vi "CalcDirection.vi"(8 "error in (no error)":errorcluster, 9 "DirectionY":i8, 10 "DirectionX":i8, 11 "Snake in":refnum<class "Snake.lvclass">) -> (0 "error out":errorcluster, 3 "Snake out":refnum<class "Snake.lvclass">)   [LabVIEW 2019, in "RT_Game.lvlib" / "Snake.lvclass"]
uses:
  Snake.lvclass
  Snake.lvclass/Snake.ctl
  Direction.ctl
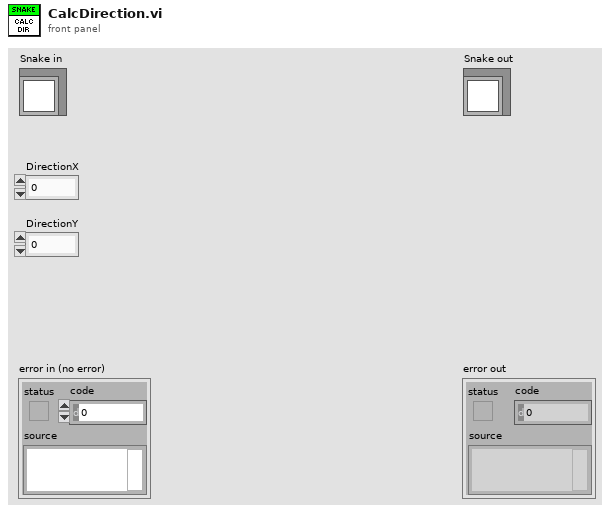
[diagram p1: front panel]
types:
  T1 = typedef "RT_Game.lvlib/Snake.lvclass/Direction.ctl" = enum16{"Up", "Left", "Down", "Right"}
  T2 = typedef "RT_Game.lvlib/Game.lvclass/Coordinate.ctl" = cluster{"x":dbl, "y":dbl}
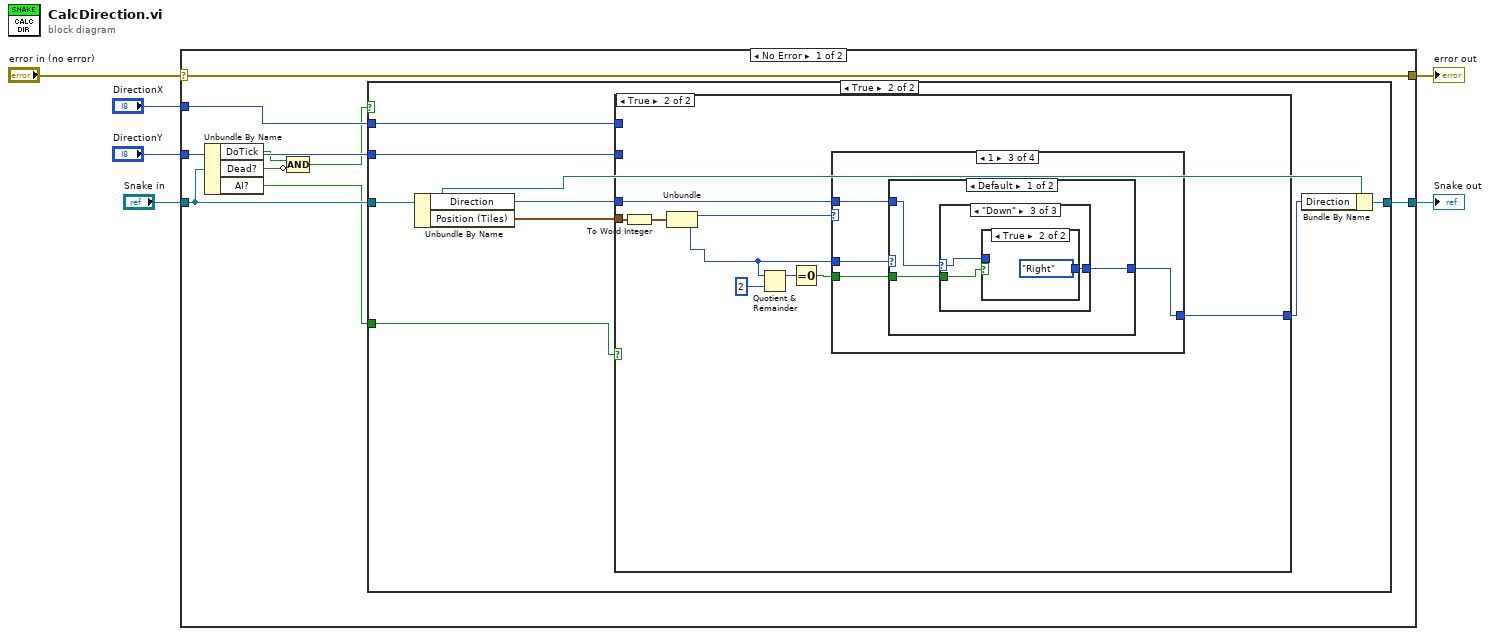
[diagram p0: block diagram]
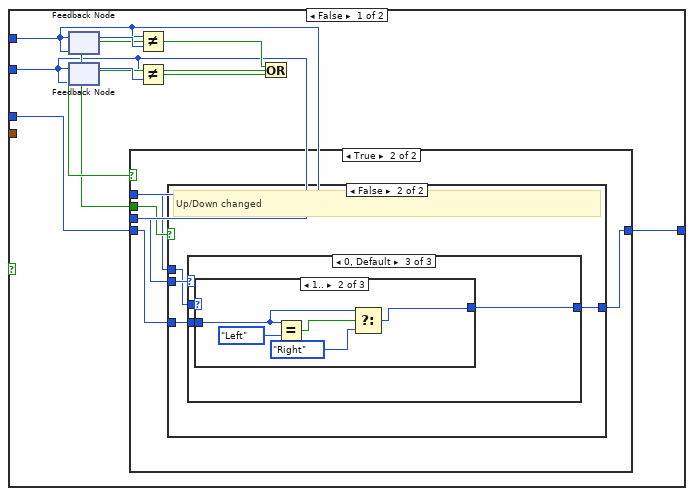
[diagram p3: hidden frame]
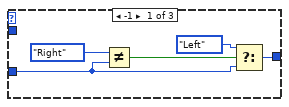
[diagram p6: hidden frame]
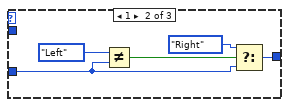
[diagram p7: hidden frame]
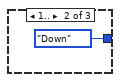
[diagram p8: hidden frame]
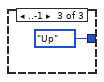
[diagram p9: hidden frame]
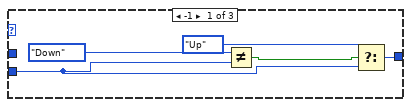
[diagram p10: hidden frame]
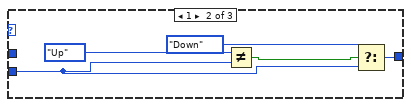
[diagram p11: hidden frame]
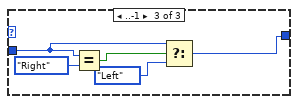
[diagram p13: hidden frame]
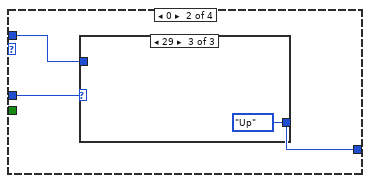
[diagram p15: hidden frame]
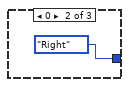
[diagram p17: hidden frame]
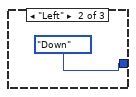
[diagram p19: hidden frame]
diagram:
  n1 = case shown="No Error" "error in (no error)" {
    selector: "error in (no error)" -> [w15 w125]
    tunnel: [w15 w125] -> w5
    tunnel: [w14 w124] -> w3
    tunnel: "Snake in" -> [w11 w124]
    tunnel: "DirectionX" -> [w13 _]
    tunnel: "DirectionY" -> [w12 _]
    frame No Error {
      n2 = Unbundle By Name(w11) -> ("DoTick"=w8:bool, "Dead?"=w10:bool, "AI?"=w7:bool)
      n3 = Compound Arithmetic op=AND(w8, invert w10) -> (w9:bool)
      n4 = case shown="True" w9 {
        tunnel: [w16 w23] -> w14
        tunnel: w13 -> [_ w21]
        tunnel: w12 -> [_ w20]
        tunnel: w11 -> [w16 w19]
        tunnel: w7 -> [_ w18]
        frame False {
        }
        frame True {
          n5 = Unbundle By Name(w19) -> ("Direction"=w24:T1, "Position (Tiles)"=w17:T2)
          n6 = case shown="True" w18 {
            tunnel: w24 -> [w28 w94]
            tunnel: [w27 w93] -> w22
            tunnel: w21 -> [w26 _]
            tunnel: w20 -> [w25 _]
            tunnel: w17 -> [_ w96]
            frame False {
              n7 = feedback #1(w26) -> (w33:i8)
              n8 = feedback-in #1(w26) -> ()
              n9 = feedback #2(w25) -> (w32:i8)
              n10 = feedback-in #2(w25) -> ()
              n11 = Not Equal?(x=w26, y=w33) -> (x != y?=w29:bool)
              n12 = Not Equal?(x=w25, y=w32) -> (x != y?=w31:bool)
              n13 = Or(x=w29, y=w31) -> (x .or. y?=w30:bool)
              n14 = case shown="True" w30 {
                tunnel: w26 -> [_ w38]
                tunnel: w25 -> [_ w35]
                tunnel: w29 -> [_ w39]
                tunnel: w28 -> [w34 w37]
                tunnel: [w34 w36] -> w27
                frame False {
                }
                frame True {
                  n15 = case shown="False" w39 {
                    tunnel: w38 -> [w43 w60]
                    tunnel: w37 -> [w42 w63]
                    tunnel: [w41 w62] -> w36
                    tunnel: w35 -> [w40 w61]
                    frame True {
                      # "Left/Right changed"
                      n16 = case shown="0, Default" w43 {
                        tunnel: [w46 w49 w55] -> w41
                        tunnel: w42 -> [w47 w50 w54]
                        tunnel: w40 -> [_ _ w56]
                        frame -1 {
                          n17 = Not Equal?(x=Direction."Right", y=w47) -> (x != y?=w45:bool)
                          n18 = Select(t=Direction."Left", s=w45, f=w47) -> (s? t:f=w46:T1)
                        }
                        frame 1 {
                          n19 = Not Equal?(x=Direction."Left", y=w50) -> (x != y?=w53:bool)
                          n20 = Select(t=Direction."Right", s=w53, f=w50) -> (s? t:f=w49:T1)
                        }
                        frame 0, Default {
                          n21 = case shown="0, Default" w56 {
                            tunnel: [w57 Direction."Down" ("Direction") Direction."Up" ("Direction")] -> w55
                            tunnel: w54 -> [w57 _ _]
                            frame 0, Default {
                            }
                            frame 1.. {
                            }
                            frame ..-1 {
                            }
                          }
                        }
                      }
                    }
                    frame False {
                      # "Up/Down changed"
                      n22 = case shown="0, Default" w61 {
                        tunnel: [w66 w69 w75] -> w62
                        tunnel: w63 -> [w67 w70 w74]
                        tunnel: w60 -> [_ _ w76]
                        frame -1 {
                          n23 = Not Equal?(x=Direction."Down", y=w67) -> (x != y?=w65:bool)
                          n24 = Select(t=Direction."Up", s=w65, f=w67) -> (s? t:f=w66:T1)
                        }
                        frame 1 {
                          n25 = Not Equal?(x=Direction."Up", y=w70) -> (x != y?=w73:bool)
                          n26 = Select(t=Direction."Down", s=w73, f=w70) -> (s? t:f=w69:T1)
                        }
                        frame 0, Default {
                          n27 = case shown="1.." w76 {
                            tunnel: [w77 w78 w83] -> w75
                            tunnel: w74 -> [w77 w80 w84]
                            frame 0, Default {
                            }
                            frame 1.. {
                              n28 = Equal?(x=w80, y=Direction."Left") -> (x = y?=w81:bool)
                              n29 = Select(t=w80, s=w81, f=Direction."Right" ("Direction")) -> (s? t:f=w78:T1)
                            }
                            frame ..-1 {
                              n30 = Equal?(x=w84, y=Direction."Right") -> (x = y?=w86:bool)
                              n31 = Select(t=w84, s=w86, f=Direction."Left" ("Direction")) -> (s? t:f=w83:T1)
                            }
                          }
                        }
                      }
                    }
                  }
                }
              }
            }
            frame True {
              n32 = To Word Integer(number=w96) -> (16bit integer=w95:cluster{"x":i16, "y":i16})
              n33 = Unbundle(w95) -> ("x"=w92:i16, "y"=w91:i16)
              n34 = Quotient & Remainder(x=w91, y=i16 2) -> (x-y*floor(x/y)=w89:i16)  [unwired: 1 out]
              n35 = Equal To 0?(x=w89) -> (x = 0?=w88:bool)
              n36 = case shown="1" w92 {
                tunnel: w94 -> [w97 w98 w105 w119]
                tunnel: [w97 w99 w106 w120] -> w93
                tunnel: w91 -> [_ w100 w107 _]
                tunnel: w88 -> [_ _ w104 _]
                frame Default {
                }
                frame 0 {
                  n37 = case shown="29" w100 {
                    tunnel: [w101 Direction."Right" ("Direction") Direction."Up" ("Direction")] -> w99
                    tunnel: w98 -> [w101 _ _]
                    frame Default {
                    }
                    frame 0 {
                    }
                    frame 29 {
                    }
                  }
                }
                frame 1 {
                  n38 = case shown="Default" w107 {
                    tunnel: [w109 w118] -> w106
                    tunnel: w105 -> [w110 w118]
                    tunnel: w104 -> [w108 _]
                    frame Default {
                      n39 = case shown="\"Down\"" w110 {
                        selector: w110 -> [w111 _ w114]
                        tunnel: [w111 Direction."Down" ("Direction") w115] -> w109
                        tunnel: w108 -> [_ _ w113]
                        frame Default {
                        }
                        frame "Left" {
                        }
                        frame "Down" {
                          n40 = case shown="True" w113 {
                            tunnel: [w116 Direction."Right" ("Direction")] -> w115
                            tunnel: w114 -> [w116 _]
                            frame False {
                            }
                            frame True {
                            }
                          }
                        }
                      }
                    }
                    frame 29 {
                      # "left"
                    }
                  }
                }
                frame 39 {
                  n41 = case shown="\"Down\"" w119 {
                    selector: w119 -> [w121 _ _]
                    tunnel: [w121 Direction."Down" ("Direction") Direction."Left" ("Direction")] -> w120
                    frame Default {
                    }
                    frame "Right" {
                    }
                    frame "Down" {
                    }
                  }
                }
              }
            }
          }
          n42 = Bundle By Name(cluster=w19, "Direction"=w22) -> (w23:refnum<class "Snake.lvclass">)
        }
      }
    }
    frame Error {
    }
  }
  "error out" <- w5
  "Snake out" <- w3
